vi "Configure Current Limit.vi"(7 "Enable OCP (T: Enable)":bool=TRUE caption="Enable OVP (T: Enable)", 8 "error in (no error)":errorcluster, 9 "Current Limit (5.0 A)":dbl=5.0 caption="Current Limit (5 A)" format="%.2f", 10 "Channel (0: 30V Channel)":T1 caption="Channel (0: +6V)" items=["30V/3A Channel", "30V/3A Channel", "5V/3A Channel"], 11 "VISA resource name":refnum<visa-resource-name>) -> (0 "error out":errorcluster, 3 "VISA resource name out":refnum<visa-resource-name>)   [LabVIEW 2020, in "Library Instrument & Equipement.lvlib" / "Library Power_Supply.lvlib" / "RIGOL DP800 Series.lvlib"]
doc: "Configures over current protection (OCP). Specify the output current limit value and the behavior of the power supply when the output current is greater than or equal to that value."
uses:
  RIGOL DP800 Series.lvlib
  Channels.ctl
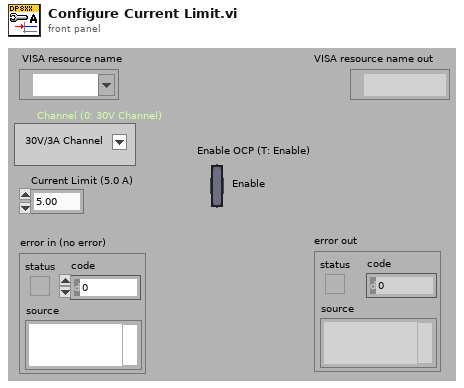
[diagram p1: front panel]
types:
  T1 = typedef "Library Instrument & Equipement.lvlib/Library Power_Supply.lvlib/RIGOL DP800 Series.lvlib/Channels.ctl" = i32
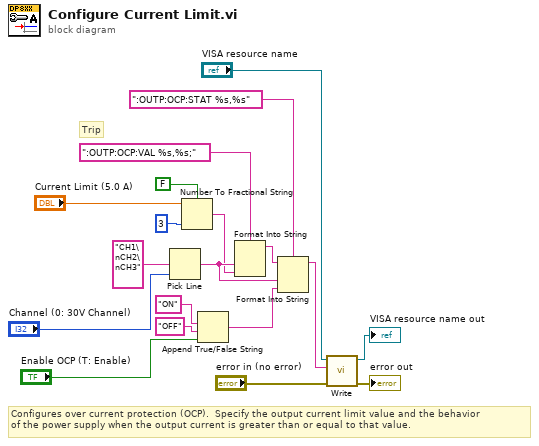
[diagram p0: block diagram]
diagram:
  # "Trip"
  # "Configures over current protection (OCP).  Specify the output current limit value and the behavior \nof the power supply when the output current is greater than or equal to that value."
  n1 = Pick Line(multi-line string="CH1\nCH2\nCH3", line index="Channel (0: 30V Channel)") -> (output string=w18:string)  [unwired: 1 in]
  n2 = Number To Fractional String(use system decimal point (T)=FALSE ("utiliser le séparateur décimal du système (V)"), number="Current Limit (5.0 A)", precision (6)=i16 3 ("précision (6)")) -> (F-format string=w8:string)  [unwired: 1 in]
  n3 = Append True/False String(1:"Enable OCP (T: Enable)", 2:"OFF", 3:"ON") -> (0:w2:string)  [unwired: 1 out]
  n4 = Format Into String(format string=":OUTP:OCP:VAL %s,%s;", w18, w8) -> (resulting string=w6:string)  [unwired: 2 in, 1 out]
  n5 = Format Into String(format string=":OUTP:OCP:STAT %s,%s", initial string=w6, w18, w2) -> (resulting string=w13:string)  [unwired: 1 in, 1 out]
  n6 = call "Write.vi"("error in (no error)"="error in (no error)", "Write Buffer (\"\")"=w13, "VISA resource name"="VISA resource name") -> ("error out"=→"error out":errorcluster, "VISA resource name out"=→"VISA resource name out":refnum<visa-resource-name>)  [unwired: 7 in]
